vi "Get Transformation Components.vi"(0 "2xN Matrix":T1=[[0.8660254037844387, -0.49999999999999994, 0.0], [0.49999999999999994, 0.8660254037844387, 0.0]]) -> (1 "xx":dbl, 2 "ty":dbl, 3 "xy":dbl, 4 "yx":dbl, 5 "yy":dbl, 6 "tx":dbl)   [LabVIEW 2023, in "Glyph Drawer.lvlib"]
uses:
  <vilib>/Analysis/Matrix/Datatypes/RealMatrix.ctl
  Glyph/Glyph Drawer.lvlib
  <vilib>/Analysis/Matrix/NI_Matrix.lvlib
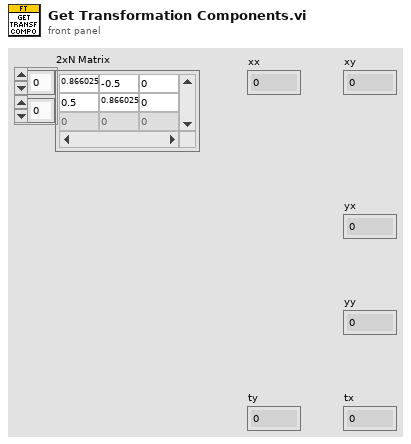
[diagram p1: front panel]
types:
  T1 = typedef "NI_Matrix.lvlib/RealMatrix.ctl" = dbl[][]
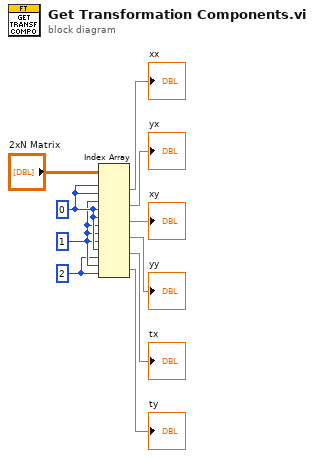
[diagram p0: block diagram]
diagram:
  w8 = 2 ("index (col)")
  w9 = 1 ("index (row)")
  w10 = 0 ("index (row)")
  n1 = Index Array(array="2xN Matrix", index (row) #1=w10, index (col) #1=w10, index (row) #2=w9, index (col) #2=w10, index (row) #3=w10, index (col) #3=w9, index (row) #4=w9, index (col) #4=w9, index (row) #5=w10, index (col) #5=w8, index (row) #6=w9, index (col) #6=w8) -> (element #1=→"xx":dbl, element #2=→"yx":dbl, element #3=→"xy":dbl, element #4=→"yy":dbl, element #5=→"tx":dbl, element #6=→"ty":dbl)
